vi "Xml_Save_Sequence.vi"(8 "error in (no error)":errorcluster, 11 "Refnum Clust":refnum<vi>) -> (0 "error out":errorcluster, 3 "XML String Out":string[](array[string]))   [LabVIEW 2024]
uses:
  controls/SEQUENCE_Inputs.ctl
  controls/EXCIT_Inputs.ctl
  controls/DATA_Inputs.ctl
  controls/TIMING_Inputs.ctl
  controls/PROCESSING_Inputs.ctl
  controls/TRAPPING_Inputs.ctl
  controls/RF_TRAPPING_Inputs.ctl
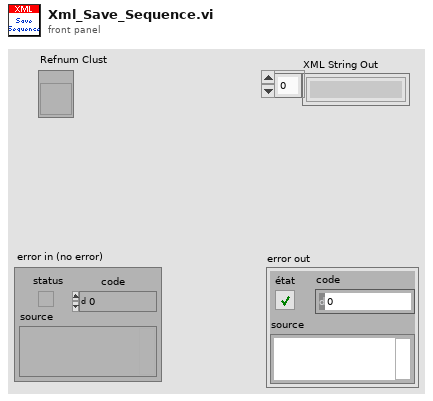
[diagram p1: front panel]
types:
  T1 = typedef "SEQUENCE_Inputs.ctl" = cluster{"EXCIT Inputs":T2, "DATA Inputs":T3, "TIMING Inputs":T4, "PROCESSING Inputs":T5, "TRAPPING Inputs":T6, "RF_TRAPPING Inputs":T7}
  T2 = typedef "EXCIT_Inputs.ctl" = cluster{"Number of Excitations":i32, "Script Text":string, "Table of Waveforms":string[]}
  T3 = typedef "DATA_Inputs.ctl" = cluster{"Record Length":i32, "Sample Rate":dbl, "Data Type":u8, "Vertical Range":dbl, "Acquisition Duration":dbl}
  T4 = typedef "TIMING_Inputs.ctl" = cluster{"Number of Acquisitions ":i16, "Number of Accumulations":i16, "Table of Waveforms":string[], "Script Text":string}
  T5 = typedef "PROCESSING_Inputs.ctl" = cluster{"Reference Mass":dbl, "Cyclotron Freq":dbl, "Magnetron Freq":dbl}
  T6 = typedef "TRAPPING_Inputs.ctl" = cluster{"Number of Channels":i32, "Init Values":dbl[], "Opening Values":dbl[], "Trapping Values":dbl[], "Emptying Values":dbl[], "Adiabatic ON":bool, "Adiabatic Duration":i32, "Adiabatic Waveforms":string[], "Ions Refill ON":bool, "Number of Ions Refills":i32}
  T7 = typedef "RF_TRAPPING_Inputs.ctl" = cluster{"Init Values":dbl[], "Opening Values":dbl[], "Trapping Values":dbl[], "Emptying Values":dbl[], "RF Trap ON":bool, "RF Accums":i32, "Number of Voltages":i32}
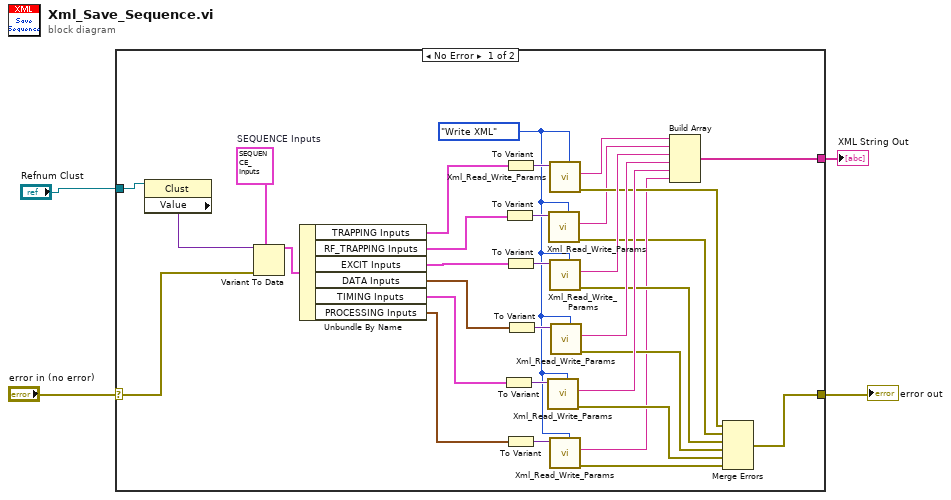
[diagram p0: block diagram]
diagram:
  n1 = case shown="No Error" "error in (no error)" {
    selector: "error in (no error)" -> [w36 w37]
    tunnel: [w34 w37] -> w3
    tunnel: [w35 _] -> w2
    tunnel: "Refnum Clust" -> [w16 _]
    frame No Error {
      w32 = T1 {"EXCIT Inputs"={"Number of Excitations"=0, "Script Text"="", "Table of Waveforms"=[]}, "DATA Inputs"={"Record Length"=0, "Sample Rate"=0.0, "Data Type"=0, "Vertical Range"=0.0, "Acquisition Duration"=0.0}, "TIMING Inputs"={"Number of Acquisitions "=0, "Number of Accumulations"=0, "Table of Waveforms"=[], "Script Text"=""}, "PROCESSING Inputs"={"Reference Mass"=0.0, "Cyclotron Freq"=0.0, "Magnetron Freq"=0.0}, "TRAPPING Inputs"={"Number of Channels"=0, "Init Values"=[], "Opening Values"=[], "Trapping Values"=[], "Emptying Values"=[], "Adiabatic ON"=FALSE, "Adiabatic Duration"=0, "Adiabatic Waveforms"=[], "Ions Refill ON"=FALSE, "Number of Ions Refills"=0}, "RF_TRAPPING Inputs"={"Init Values"=[0.0, 1.0, 1.0, 0.0], "Opening Values"=[0.0, -4.0, 1.0, 0.0], "Trapping Values"=[0.0, 1.0, 1.0, 0.0], "Emptying Values"=[0.0, 1.0, -7.0, 0.0], "RF Trap ON"=FALSE, "RF Accums"=1, "Number of Voltages"=4}}  # SEQUENCE Inputs
      w8 = enum16{"Read XML", "Set", "Get", "Write XML"}."Write XML" ("Command")
      n2 = property class="Clust"(reference=w16) -> ("Value"=w15:variant)  [unwired: 1 in, 2 out]
      n3 = Variant To Data(error in=w36, type=w32, Variant=w15) -> (data=w31:T1)  [unwired: 1 out]
      n4 = Unbundle By Name(w31) -> ("TRAPPING Inputs"=w10:T6, "RF_TRAPPING Inputs"=w7:T7, "EXCIT Inputs"=w23:T2, "DATA Inputs"=w22:T3, "TIMING Inputs"=w21:T4, "PROCESSING Inputs"=w13:T5)
      n5 = To Variant(anything=w21) -> (Variant=w28:variant)
      n6 = To Variant(anything=w7) -> (Variant=w9:variant)
      n7 = To Variant(anything=w10) -> (Variant=w33:variant)
      n8 = To Variant(anything=w23) -> (Variant=w30:variant)
      n9 = To Variant(anything=w13) -> (Variant=w14:variant)
      n10 = To Variant(anything=w22) -> (Variant=w29:variant)
      n11 = call "Xml_Read_Write_Params.vi"("Variant"=w28, "Command"=w8) -> ("XML String Out"=w27:string, "error out"=w20:errorcluster)  [unwired: 5 in, 1 out]
      n12 = call "Xml_Read_Write_Params.vi"("Variant"=w9, "Command"=w8) -> ("XML String Out"=w6:string, "error out"=w5:errorcluster)  [unwired: 5 in, 1 out]
      n13 = call "Xml_Read_Write_Params.vi"("Variant"=w33, "Command"=w8) -> ("XML String Out"=w24:string, "error out"=w17:errorcluster)  [unwired: 5 in, 1 out]
      n14 = call "Xml_Read_Write_Params.vi"("Variant"=w30, "Command"=w8) -> ("XML String Out"=w25:string, "error out"=w18:errorcluster)  [unwired: 5 in, 1 out]
      n15 = call "Xml_Read_Write_Params.vi"("Variant"=w14, "Command"=w8) -> ("XML String Out"=w11:string, "error out"=w12:errorcluster)  [unwired: 5 in, 1 out]
      n16 = call "Xml_Read_Write_Params.vi"("Variant"=w29, "Command"=w8) -> ("XML String Out"=w26:string, "error out"=w19:errorcluster)  [unwired: 5 in, 1 out]
      n17 = Build Array(w24, w6, w25, w26, w27, w11) -> (w35:string[])
      n18 = Merge Errors(w17, w5, w18, w19, w20, w12) -> (w34:errorcluster)
    }
    frame Error {
    }
  }
  "error out" <- w3
  "XML String Out" <- w2
